vi "HelloWorld_cmd.vi"() -> ()   [LabVIEW 2018]
uses:
  <vilib>/Utility/sysdir.llb/System Directory Type.ctl
  <vilib>/ptbypt/NI_PtbyPt.lvlib
panel:
  out "Mean Execution Time (s)":dbl
  out "Execution Time":dbl(graph)
  out "Output":string
  out "Error Out":errorcluster
  in  "Name":string="World"
  in  "stop":bool
  # "This VI Demonstrates using the System Exec VI to call a python function and benchmarks its execution time for comparison with other methods of communicating with Python in LabVIEW.\n\n1. Enter your name in the Name input to be personally greeted\n2. Run the VI"
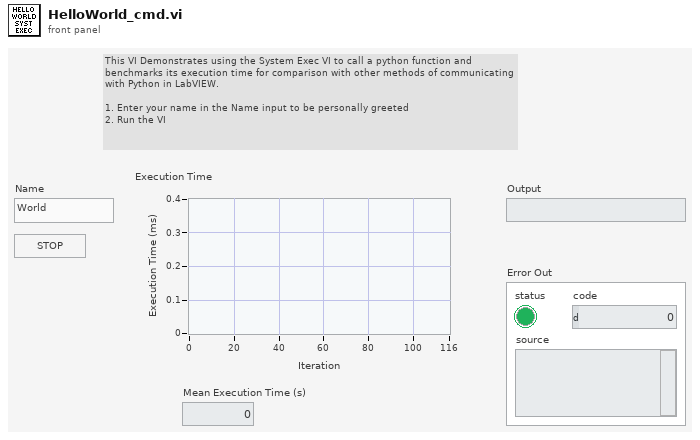
[diagram p1: front panel]
types:
  T1 = typedef "System Directory Type.ctl" = i32
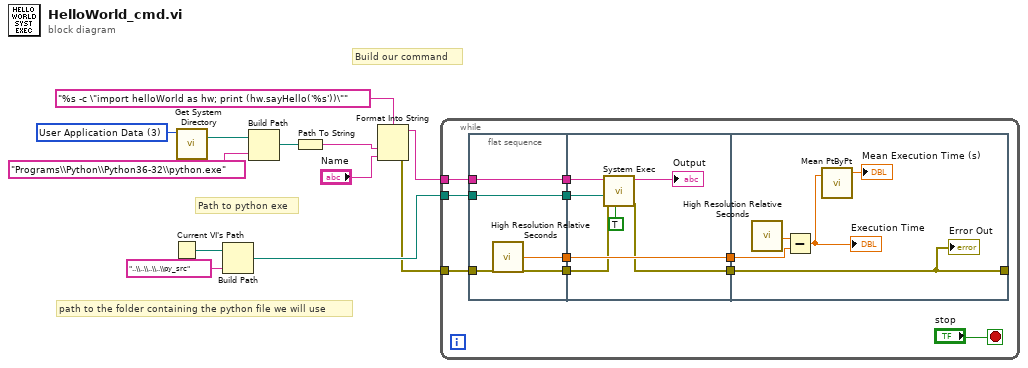
[diagram p0: block diagram]
diagram:
  w12 = T1 3 items=["User Home"=0, "User Desktop"=1, "User Documents"=2, "User Application Data"=3, "User Preferences"=4, "User Temporary"=5, "Public Documents"=6, "Public Application Data"=7, "Public Preferences"=8, "Public Cache"=13, "System Core Libraries"=9, "System Installed Libraries"=10, "Application Files"=11, "Boot Volume Root"=12] ("system directory type")
  # "Path to python exe"
  # "Build our command"
  # "path to the folder containing the python file we will use"
  n1 = Current VI's Path() -> (path=w11:path)
  n2 = call <vilib>:"Get System Directory.vi"("system directory type"=w12) -> ("system directory"=w8:path)  [unwired: 10 in]
  n3 = Build Path(base path=w11, name or relative path="..\\..\\..\\..\\py_src") -> (appended path=w9:path)
  n4 = Build Path(base path=w8, name or relative path="Programs\\Python\\Python36-32\\python.exe") -> (appended path=w6:path)
  n5 = Path To String(path=w6) -> (string=w4:string)
  n6 = Format Into String(format string="%s -c \"import helloWorld as hw; print (hw.sayHello('%s'))\"", w4, "Name") -> (resulting string=w1:string, error out=w2:errorcluster)  [unwired: 2 in]
  n7 = while {
    tunnel: w9 -> [w22]
    tunnel: w1 -> [w16]
    tunnel: w2 -> [w13]
    stop <- "stop" stop-if-true
    n8 = flat-sequence {
      tunnel: w22 -> [w26]
      tunnel: [w26] -> w20
      tunnel: [w25] -> w19
      tunnel: [w24] -> w17
      tunnel: w16 -> [w24]
      tunnel: [w23] -> w14
      tunnel: w13 -> [w23]
      tunnel: [w28] -> w21
      tunnel: w20 -> [w33]
      tunnel: w19 -> [w32]
      tunnel: [w32] -> w18
      tunnel: w17 -> [w30]
      tunnel: w14 -> [w27]
      tunnel: [w34] -> _
      tunnel: w21 -> [w34]
      tunnel: w18 -> [w37]
      frame #0 {
        n9 = call <vilib>:"High Resolution Relative Seconds.vi"() -> ("relative seconds"=w25:dbl)
      }
      frame #1 {
        n10 = call <vilib>:"System Exec.vi"("run minimized? (F)"=TRUE, "error in (no error)"=w27, "working directory"=w33, "command line"=w30) -> ("error out"=w28:errorcluster, "standard output"=→"Output":string)  [unwired: 4 in, 2 out]
      }
      frame #2 {
        n11 = call <vilib>:"High Resolution Relative Seconds.vi"() -> ("relative seconds"=w38:dbl)
        n12 = Subtract(x=w38, y=w37) -> (x-y=w36:dbl)
        "Execution Time" <- w36
        n13 = call <vilib>:"Mean PtByPt.vi"("x"=w36) -> ("mean"=→"Mean Execution Time (s)":dbl)  [unwired: 3 in, 1 out]
        "Error Out" <- w34
      }
    }
  }
